vi "Test syslog time.vi"() -> ()   [LabVIEW 2021]
uses:
  <vilib>/CIF Foundation/CIF Utilities/Time/Time_CIF_U.lvlib
  src/CIFUtilities/CIFLogs/CIFLogs.lvlib
  src/CIFUtilities/CIFLogs/Typedef/Message Type.ctl
panel:
  out "size (bytes)":i64
  out "Last Timestamp":string
  out "concatenated string":string
  out "error out":errorcluster
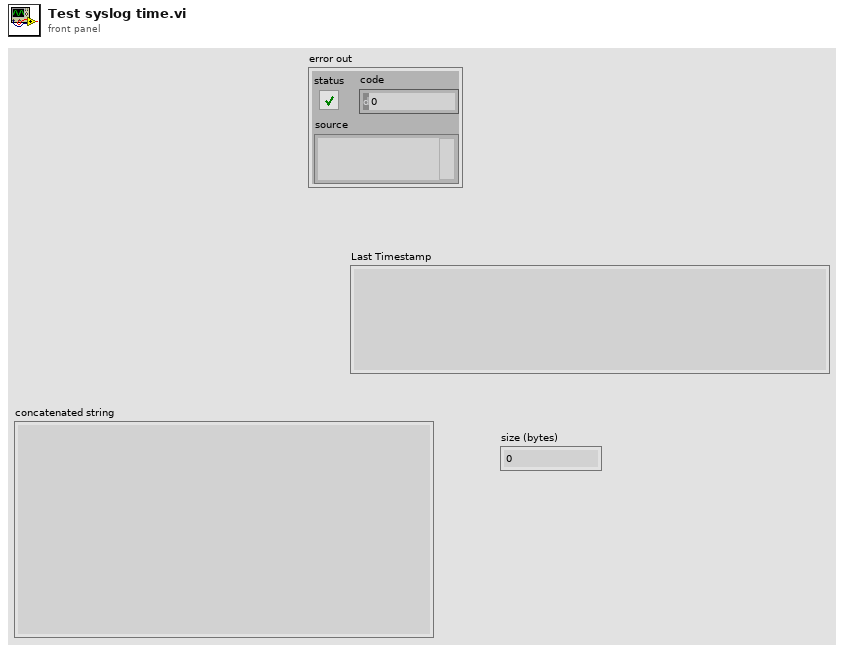
[diagram p1: front panel]
types:
  T1 = typedef "CIFLogs.lvlib/Message Type.ctl" = enum16{"Error", "Information", "Print Terminal", "Configuration"}
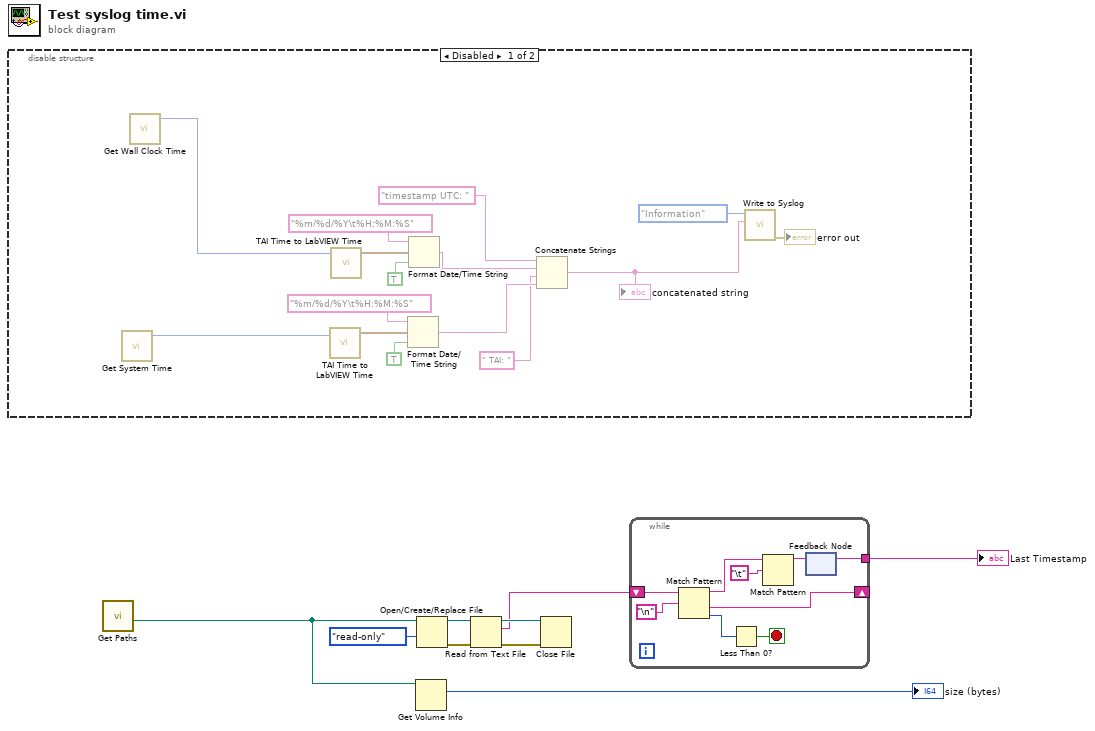
[diagram p0: block diagram]
diagram:
  n1 = disable-structure shown="Disabled" {
    frame Disabled {
      n2 = call <vilib>:"Get System Time.vi"() -> ("Time (ns)"=w11:i64)  [unwired: 5 in]
      n3 = call <vilib>:"Get Wall Clock Time.vi"() -> ("Time (ns)"=w10:i64)  [unwired: 5 in]
      n4 = call <vilib>:"TAI Time to LabVIEW Time.vi"("TAI Time (ns)"=w11) -> ("LabVIEW Time (s)"=w20:timestamp)  [unwired: 4 in]
      n5 = call <vilib>:"TAI Time to LabVIEW Time.vi"("TAI Time (ns)"=w10) -> ("LabVIEW Time (s)"=w21:timestamp)  [unwired: 4 in]
      n6 = Format Date/Time String(time format string (%c)="%m/%d/%Y\t%H:%M:%S", seconds (now)=w20, UTC format=TRUE) -> (date/time string=w16:string)
      n7 = Format Date/Time String(time format string (%c)="%m/%d/%Y\t%H:%M:%S", seconds (now)=w21, UTC format=TRUE) -> (date/time string=w17:string)
      n8 = Concatenate Strings("timestamp UTC: " ("string"), w17, " TAI: " ("string"), w16) -> (w13:string)
      "concatenated string" <- w13
      n9 = call "Write to Syslog.vi"("message"=w13, "CIF Message Type"=Message_Type."Information") -> ("error out"=→"error out":errorcluster)  [unwired: 9 in]
    }
    frame Enabled {
    }
  }
  n10 = call "Get Paths.vi"() -> ("Info Log"=w4:path)  [unwired: 9 in, 2 out]
  n11 = Get Volume Info(11:w4) -> (2:→"size (bytes)":i64)  [unwired: 1 in, 5 out]
  n12 = Open/Create/Replace File(file path (use dialog)=w4, access (0:read/write)=enum16{"read/write", "read-only", "write-only"}."read-only") -> (refnum out=w8:refnum<file>, error out=w7:errorcluster)  [unwired: 4 in, 1 out]
  n13 = Read from Text File(file (use dialog)=w8, error in=w7) -> (refnum out=w9:refnum<file>, text=w3:string, error out=w6:errorcluster)  [unwired: 2 in, 1 out]
  n14 = Close File(refnum=w9, error in=w6) -> ()  [unwired: 2 out]
  n15 = while {
    shift-right: [w32] -> _
    shift-left: w3 -> [w33]
    tunnel: [w25] -> w1
    stop <- w30 stop-if-true
    n16 = Match Pattern(string=w33, regular expression="\n") -> (before substring=w29:string, after substring=w32:string, offset past match=w31:i32)  [unwired: 1 in, 1 out]
    n17 = Less Than 0?(x=w31) -> (x < 0?=w30:bool)
    n18 = Match Pattern(string=w29, regular expression="\t") -> (before substring=w26:string)  [unwired: 1 in, 3 out]
    n19 = feedback-in #1(w26) -> ()
    n20 = feedback #1() -> (w25:string)  [unwired: 1 in]
  }
  "Last Timestamp" <- w1
